vi "SRV_Get OS Version.vi"(11 "error in (no error)":errorcluster, 12 "Min Version (6: Vista)":dbl=6.0) -> (8 "Operating System:Version Number":string, 10 "Equal or Newer Version?":bool, 15 "error out":errorcluster)   [LabVIEW 2009]
doc: "Returns the Windows operating system version number (see \"http://msdn.microsoft.com/en-us/library/windows/desktop/ms724832(v=vs.85).aspx\" for table of system version numbers). \n\nThe VI also checks if the operating system is equal to or newer than the version specified in the Min Version input.\n\n\nAuthor: Mike Schultz"
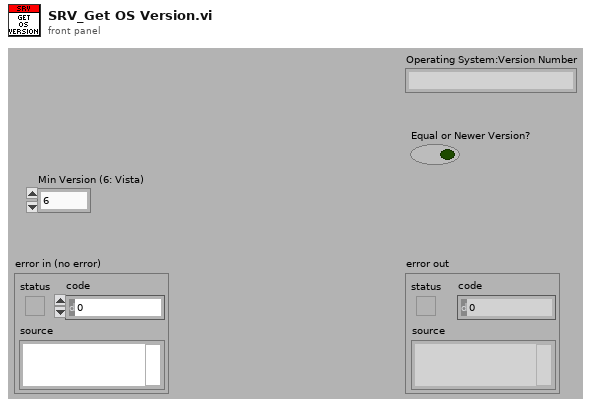
[diagram p1: front panel]
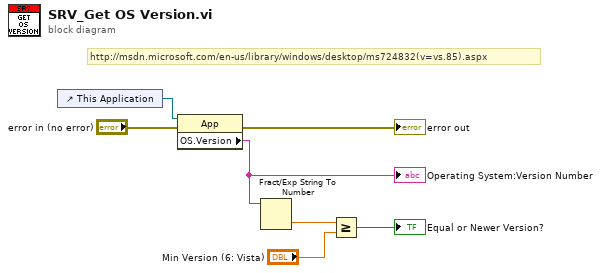
[diagram p0: block diagram]
diagram:
  # "http://msdn.microsoft.com/en-us/library/windows/desktop/ms724832(v=vs.85).aspx"
  n1 = control-ref of="This Application"() -> (w3:refnum<vi>)
  n2 = property class="App"(reference=w3, error in="error in (no error)") -> (error out=→"error out":errorcluster, "OS.Version"=w4:string)  [unwired: 1 out]
  "Operating System:Version Number" <- w4
  n3 = Fract/Exp String To Number(string=w4) -> (number=w5:dbl)  [unwired: 3 in, 1 out]
  n4 = Greater Or Equal?(x=w5, y="Min Version (6: Vista)") -> (x >= y?=→"Equal or Newer Version?":bool)
